vi "Script_Save.vi"(1 "Config Cluster in":T1, 5 "Extension":string="*.rtts", 7 "Save/SaveAs(Save= True)":bool, 9 "Script name":string, 11 "error in":errorcluster, 12 "Working Script":path) -> (3 "Config Cluster out":T1, 4 "Tree Control out":refnum<vi>, 8 "Cancelled":bool, 10 "Script name out":string, 14 "Working Script out":path, 15 "error out":errorcluster)   [LabVIEW 2011]
uses:
  Config cluster.ctl
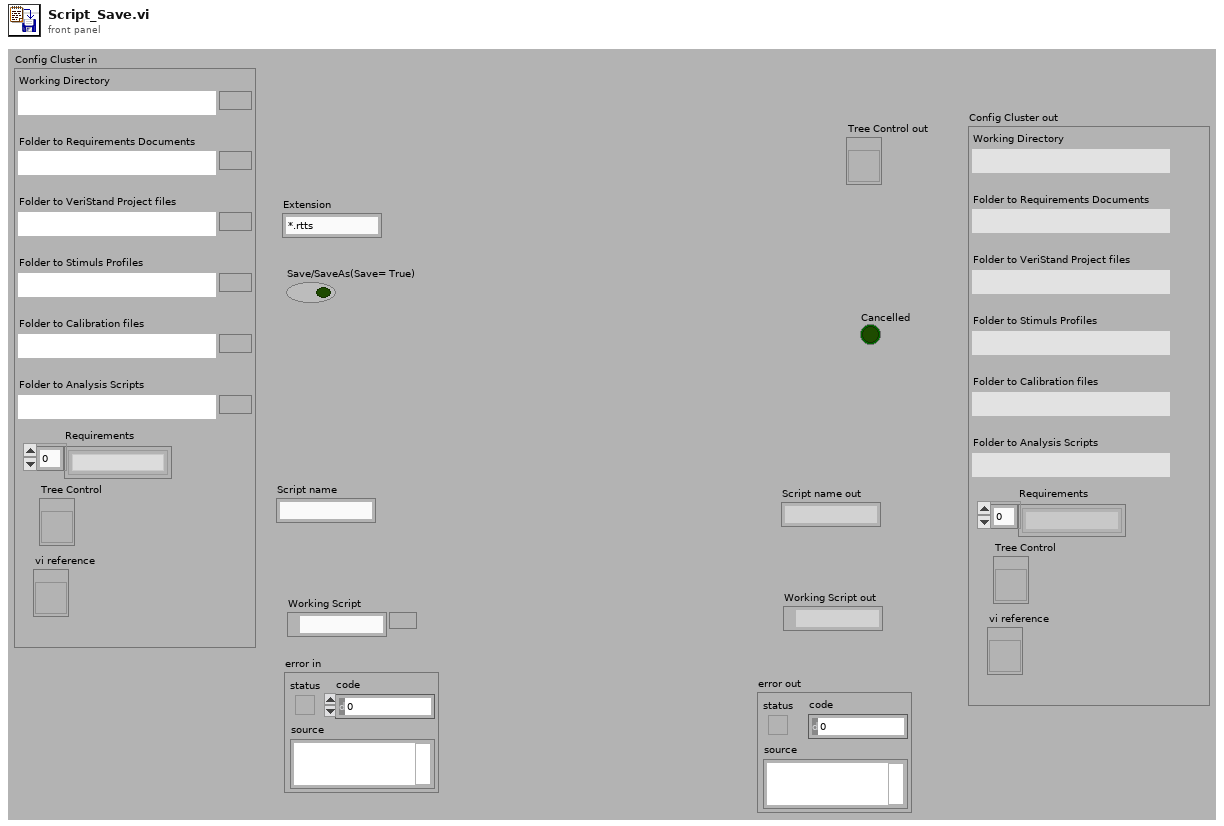
[diagram p1: front panel]
types:
  T1 = typedef "Config cluster.ctl" = cluster{"Working Directory":path, "Folder to Requirements Documents":path, "Folder to VeriStand Project files":path, "Folder to Stimuls Profiles":path, "Folder to Calibration files":path, "Folder to Analysis Scripts":path, "Requirements":string[], "Tree Control":refnum<vi>, "vi reference":refnum<vi>}
  T2 = enum16{"open", "replace", "create", "open or create", "replace or create", "replace or create with confirmation"}
  T3 = typedef "ScriptStepTypeDef.ctl" = cluster{"Indent Level":i32, "Tag":string, "Step component":string, "Req":string, "Parent Tag":string, "Symbol Index":i32}
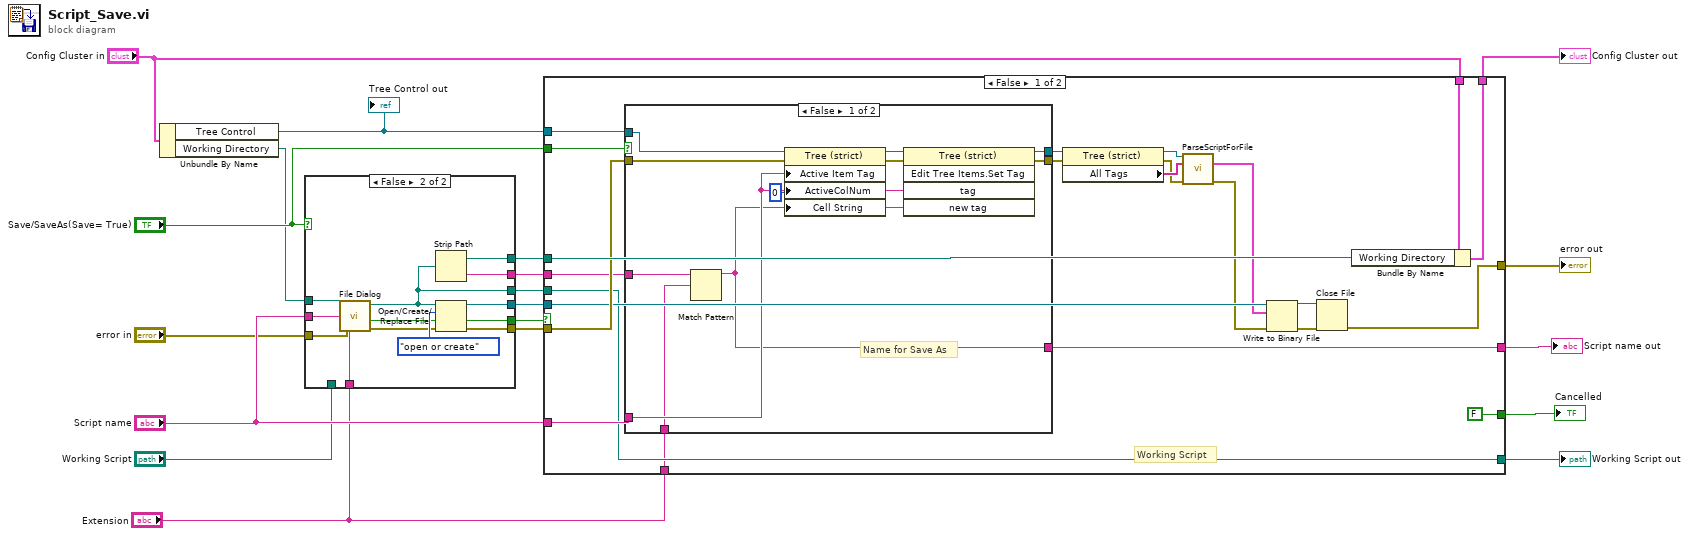
[diagram p0: block diagram]
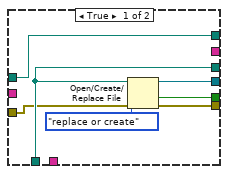
[diagram p4: hidden frame]
diagram:
  n1 = Unbundle By Name("Config Cluster in") -> ("Tree Control"=w4:refnum<vi>, "Working Directory"=w2:path)
  "Tree Control out" <- w4
  n2 = case shown="False" "Save/SaveAs(Save= True)" {
    tunnel: [w25 w37] -> w6
    tunnel: [w24 w36] -> w7
    tunnel: w2 -> [w22 w35]
    tunnel: [w23 w33] -> w11
    tunnel: [w22 w32] -> w12
    tunnel: [_ w31] -> w13
    tunnel: "Working Script" -> [w21 _]
    tunnel: [w21 w30] -> w17
    tunnel: "error in" -> [w20 w29]
    tunnel: "Script name" -> [_ w28]
    tunnel: "Extension" -> [_ w27]
    frame True {
      n3 = Open/Create/Replace File(file path (use dialog)=w21, error in=w20, operation (0:open)=T2."replace or create") -> (refnum out=w24:refnum<file>, cancelled=w23:bool, error out=w25:errorcluster)  [unwired: 3 in]
    }
    frame False {
      n4 = call "File Dialog"("start path"=w35, "default name"=w28, "error in"=w29, "pattern (all files)"=w27) -> ("selected path"=w30:path, "cancelled"=w33:bool, "error out"=w34:errorcluster)  [unwired: 8 in, 1 out]
      n5 = Strip Path(path=w30) -> (stripped path=w32:path, name=w31:string)
      n6 = Open/Create/Replace File(file path (use dialog)=w30, error in=w34, operation (0:open)=T2."open or create") -> (refnum out=w36:refnum<file>, error out=w37:errorcluster)  [unwired: 3 in, 1 out]
    }
  }
  n7 = case shown="False" w11 {
    selector: w11 -> [_ w76]
    tunnel: w6 -> [w52 _]
    tunnel: w7 -> [w51 _]
    tunnel: "Save/SaveAs(Save= True)" -> [w61 _]
    tunnel: [w48 _] -> w8
    tunnel: "Script name" -> [w60 w78]
    tunnel: [w59 w78] -> w9
    tunnel: "Config Cluster in" -> [w58 w79]
    tunnel: [w57 w79] -> w10
    tunnel: w12 -> [w56 _]
    tunnel: w13 -> [w47 _]
    tunnel: w4 -> [w55 _]
    tunnel: [w46 w77] -> w14
    tunnel: w17 -> [w46 w77]
    tunnel: [FALSE w76] -> w5
    tunnel: "Extension" -> [w39 _]
    frame False {
      # "Working Script"
      n8 = case shown="False" w61 {
        tunnel: [w69 w73] -> w53
        tunnel: w60 -> [w68 w75]
        tunnel: [w67 w75] -> w59
        tunnel: w55 -> [w66 w74]
        tunnel: [w65 w74] -> w54
        tunnel: w52 -> [w64 w73]
        tunnel: w47 -> [w63 _]
        tunnel: w39 -> [w62 _]
        frame False {
          # "Name for Save As"
          n9 = Match Pattern(string=w63, regular expression=w62) -> (before substring=w67:string)  [unwired: 1 in, 3 out]
          n10 = property class="Tree (strict)"(reference=w66, error in=w64, "Active Item Tag"=w68, "ActiveColNum"=0 ("Active Cell:Active Column Number"), "Cell String"=w67) -> (reference out=w71:refnum<vi>, error out=w70:errorcluster)
          n11 = invoke class="Tree (strict)" method="Edit Tree Items.Set Tag"(reference=w71, error in=w70, "tag"=w68, "new tag"=w67) -> (reference out=w65:refnum<vi>, error out=w69:errorcluster)  [unwired: 1 in, 3 out]
        }
        frame True {
        }
      }
      n12 = property class="Tree (strict)"(reference=w54, error in=w53) -> (reference out=w44:refnum<vi>, error out=w40:errorcluster, "All Tags"=w43:string[])
      n13 = call "ParseScriptForFile.vi"("Tree Ref in"=w44, "Script Array"=w43, "error in"=w40) -> ("Script Steps"=w42:T3[], "error out"=w41:errorcluster)  [unwired: 10 in, 1 out]
      n14 = Write to Binary File(file (use dialog)=w51, data=w42, error in=w41) -> (refnum out=w49:refnum<file>, error out=w50:errorcluster)  [unwired: 3 in, 1 out]
      n15 = Close File(refnum=w49, error in=w50) -> (error out=w48:errorcluster)  [unwired: 1 out]
      n16 = Bundle By Name(cluster=w58, "Working Directory"=w56) -> (w57:T1)
    }
    frame True {
    }
  }
  "Working Script out" <- w14
  "Config Cluster out" <- w10
  "Script name out" <- w9
  "error out" <- w8
  "Cancelled" <- w5
